vi "PH_BlackBox.read DB.vi"(1 "BB Instance":string, 5 "error in (no error)":errorcluster) -> (14 "Recipient":string, 15 "#":i32, 16 "Caption Move":string, 17 "Caption Out":string, 18 "Caption In":string, 19 "error out":errorcluster)   [LabVIEW 2014, in "PH_BlackBox.lvlib"]
uses:
  PH_BlackBox.lvlib
  PH_Basics/PH_Common/PH_Common.lvlib
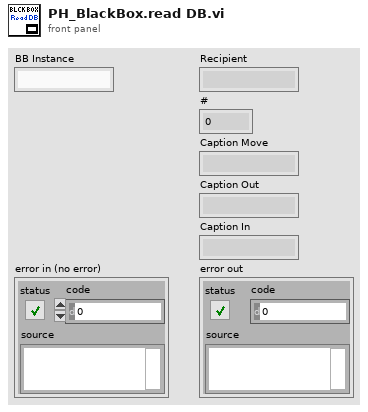
[diagram p1: front panel]
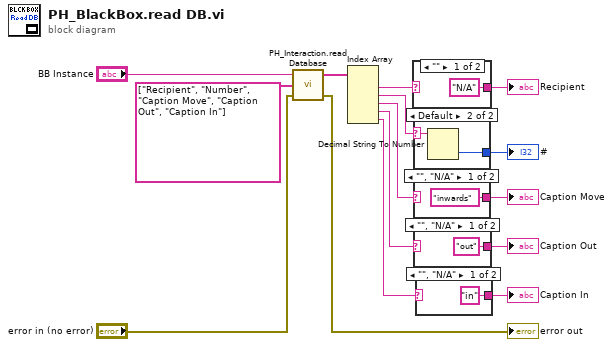
[diagram p0: block diagram]
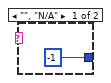
[diagram p2: hidden frame]
diagram:
  n1 = call "PH_Interaction.read Database.vi"("error in (no error)"="error in (no error)", "Strings to search for"=string[] ["Recipient", "Number", "Caption Move", "Caption Out", "Caption In"], "DB Entry to read"="BB Instance") -> ("error out"=→"error out":errorcluster, "Values"=w5:string[])  [unwired: 1 in]
  n2 = Index Array(array=w5) -> (element #1=w6:string, element #2=w14:string, element #3=w8:string, element #4=w9:string, element #5=w10:string)  [unwired: 5 in]
  n3 = case shown="\"\"" w6 {
    selector: w6 -> [_ w17]
    tunnel: ["N/A" w17] -> w7
    frame "" {
    }
    frame Default {
    }
  }
  "Recipient" <- w7
  n4 = case shown="Default" w14 {
    selector: w14 -> [_ w20]
    tunnel: [-1 w19] -> w15
    frame "", "N/A" {
    }
    frame Default {
      n5 = Decimal String To Number(string=w20) -> (number=w19:i32)  [unwired: 2 in, 1 out]
    }
  }
  "#" <- w15
  n6 = case shown="\"\", \"N/A\"" w8 {
    selector: w8 -> [_ w22]
    tunnel: ["inwards" w22] -> w11
    frame "", "N/A" {
    }
    frame Default {
    }
  }
  "Caption Move" <- w11
  n7 = case shown="\"\", \"N/A\"" w9 {
    selector: w9 -> [_ w24]
    tunnel: ["out" w24] -> w12
    frame "", "N/A" {
    }
    frame Default {
    }
  }
  "Caption Out" <- w12
  n8 = case shown="\"\", \"N/A\"" w10 {
    selector: w10 -> [_ w26]
    tunnel: ["in" w26] -> w13
    frame "", "N/A" {
    }
    frame Default {
    }
  }
  "Caption In" <- w13
